vi "QTrkAlt.vi"() -> ()   [LabVIEW 2011]
uses:
  jtrkd-labview-nt.dll
panel:
  in  "ZLUT Settings":T1={"ZLUT MinRadius"=5.0, "ZLUT MaxRadius"=50.0, "ZLUT AngularSteps"=64}
  in  "1D Cross Correlation Settings":T2={"XCOR Profile Length"=128, "XCOR Profile Width"=32, "XCOR Iterations"=2}
  in  "QTrk Main Settings":T3={"Image width"=150, "Image height"=150, "Number of threads (CPU based)"=-1, "Max Queue Size"=200}
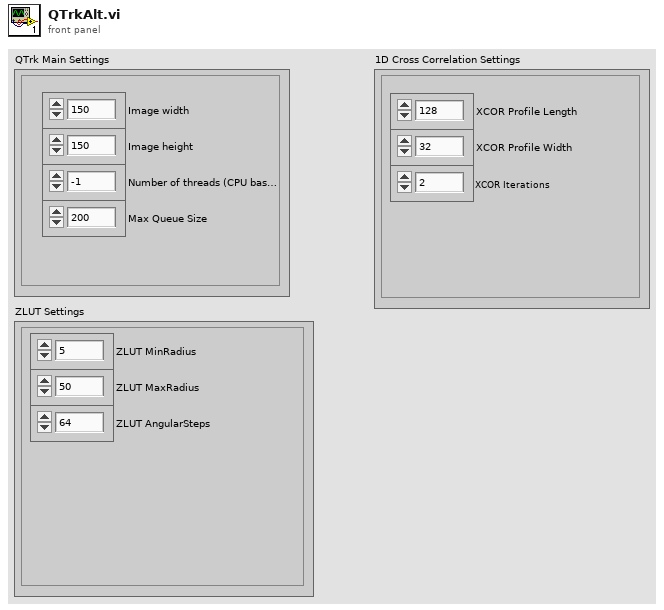
[diagram p1: front panel]
types:
  T1 = cluster{"ZLUT MinRadius":sgl, "ZLUT MaxRadius":sgl, "ZLUT AngularSteps":i32}
  T2 = cluster{"XCOR Profile Length":i32, "XCOR Profile Width":i32, "XCOR Iterations":i32}
  T3 = cluster{"Image width":i32, "Image height":i32, "Number of threads (CPU based)":i32, "Max Queue Size":i32}
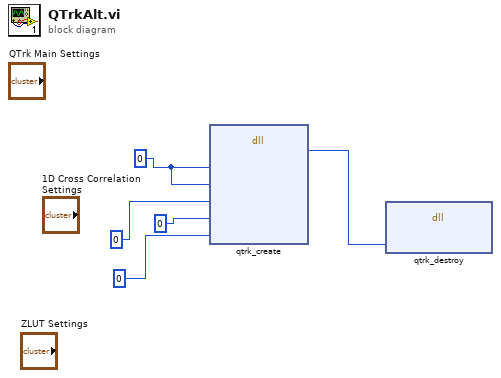
[diagram p0: block diagram]
diagram:
  w1 = 0 ("startNow")
  n1 = dll-call lib="F:/dev/jtrk/bin/jtrkd-labview-nt.dll" fn="qtrk_create"("cfg_main"=w1, "cfg_xcor"=w1, "cfg_qi"=0 ("startNow"), "cfg_zlut"=0 ("startNow"), "startNow"=0) -> ("return type"=w5:u64)  [unwired: 8 in, 2 out]
  n2 = dll-call lib="F:/dev/jtrk/bin/jtrkd-labview-nt.dll" fn="qtrk_destroy"("tracker"=w5) -> ()  [unwired: 5 in, 2 out]
